vi "Close References.vi"(8 "error in":errorcluster, 11 "input cluster":T1) -> (0 "error out":errorcluster)   [LabVIEW 2020]
doc: "This VI closes the references for all controls and indicators."
uses:
  Controls/Controls-Indicators References.ctl
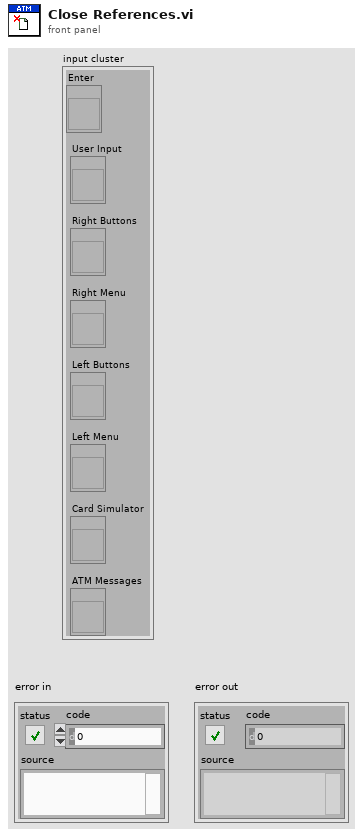
[diagram p1: front panel]
types:
  T1 = typedef "Controls-Indicators References.ctl" = cluster{"Enter":refnum<vi>, "User Input":refnum<vi>, "Right Buttons":refnum<vi>, "Right Menu":refnum<vi>, "Left Buttons":refnum<vi>, "Left Menu":refnum<vi>, "Card Simulator":refnum<vi>, "ATM Messages":refnum<vi>}
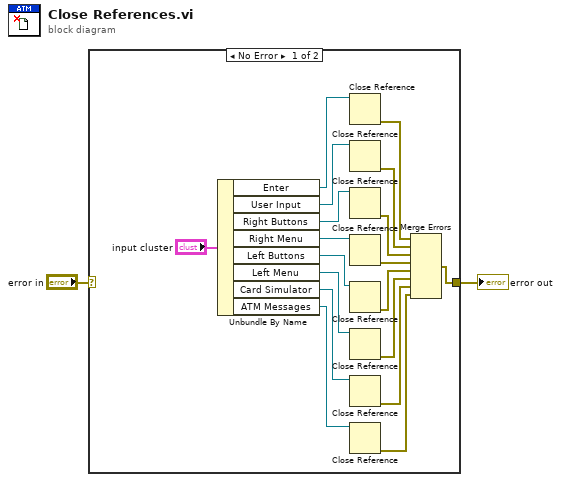
[diagram p0: block diagram]
diagram:
  n1 = case shown="No Error" "error in" {
    selector: "error in" -> [_ w21]
    tunnel: [w3 w21] -> w2
    frame No Error {
      n2 = Unbundle By Name("input cluster") -> ("Enter"=w5:refnum<vi>, "User Input"=w6:refnum<vi>, "Right Buttons"=w7:refnum<vi>, "Right Menu"=w8:refnum<vi>, "Left Buttons"=w9:refnum<vi>, "Left Menu"=w10:refnum<vi>, "Card Simulator"=w11:refnum<vi>, "ATM Messages"=w12:refnum<vi>)
      n3 = Close Reference(reference=w5) -> (error out=w13:errorcluster)  [unwired: 1 in]
      n4 = Close Reference(reference=w6) -> (error out=w14:errorcluster)  [unwired: 1 in]
      n5 = Close Reference(reference=w7) -> (error out=w15:errorcluster)  [unwired: 1 in]
      n6 = Close Reference(reference=w8) -> (error out=w16:errorcluster)  [unwired: 1 in]
      n7 = Close Reference(reference=w9) -> (error out=w17:errorcluster)  [unwired: 1 in]
      n8 = Close Reference(reference=w10) -> (error out=w18:errorcluster)  [unwired: 1 in]
      n9 = Close Reference(reference=w11) -> (error out=w19:errorcluster)  [unwired: 1 in]
      n10 = Close Reference(reference=w12) -> (error out=w20:errorcluster)  [unwired: 1 in]
      n11 = Merge Errors(w13, w14, w15, w16, w17, w18, w19, w20) -> (w3:errorcluster)
    }
    frame Error {
    }
  }
  "error out" <- w2
